vi "DeadbandJoystick.vi"(11 "SpeedInput":dbl) -> (3 "SpeedOutput":dbl)   [LabVIEW 2017]
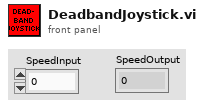
[diagram p1: front panel]
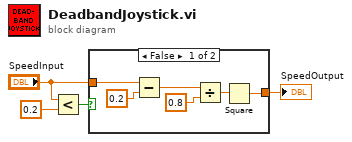
[diagram p0: block diagram]
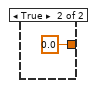
[diagram p2: hidden frame]
diagram:
  n1 = Less?(x="SpeedInput", y=0.2) -> (x < y?=w3:bool)
  n2 = case shown="False" w3 {
    tunnel: "SpeedInput" -> [w10 _]
    tunnel: [w5 0.0] -> w1
    frame False {
      n3 = Subtract(x=w10, y=0.2) -> (x-y=w8:dbl)
      n4 = Divide(x=w8, y=0.8) -> (x/y=w6:dbl)
      n5 = Square(x=w6) -> (x^2=w5:dbl)
    }
    frame True {
    }
  }
  "SpeedOutput" <- w1
